vi "Chunk by Time.vi"(9 "Time Range (ns)":i64 format="%.0e", 10 "Max Frames":i32=1, 11 "Bytes in":u8[](array[numeric])) -> (2 "Chunks":T1[](array[typedef]), 3 "Bytes out":u8[](array[numeric]))   [LabVIEW 2021, in "pcap_Parse_Build_CIF.lvclass"]
doc: "Update all timestamps in the pcap bytestream. This will automatically detect if a global header is present and will work on both full pcap streams to/from disk and pcap packets to/from FIFO. If no global header is found it will default to CIF channel format (little endian, ns timestamp)."
uses:
  pcap_Parse_Build_CIF.lvclass
  Typedef/Chunk.ctl
  pcap_Parse_Build_CIF.lvclass/pcap_Parse_Build_CIF.ctl
  Parse/Unflatten Packet Header.vi
  Add Error.vi
  <vilib>/CIF Foundation/CIF Utilities/DataTypes/Flatten Unflatten/Unflatten U32.vi
  <vilib>/CIF Foundation/CIF Utilities/Errors/Append Error Location.vi
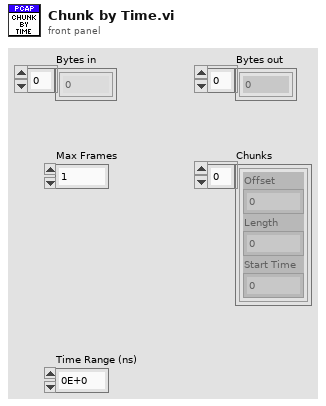
[diagram p1: front panel]
types:
  T1 = typedef "pcap_Parse_Build_CIF.lvclass/Chunk.ctl" = cluster{"Offset":i32, "Length":u32, "Start Time":i64}
  T2 = typedef "pcap_Parse_Build_CIF.lvclass/Packet Header.ctl" = cluster{"Timestamp (s)":u32, "Timestamp (ns)":u32, "Inc Length":u32, "Orig Length":u32}
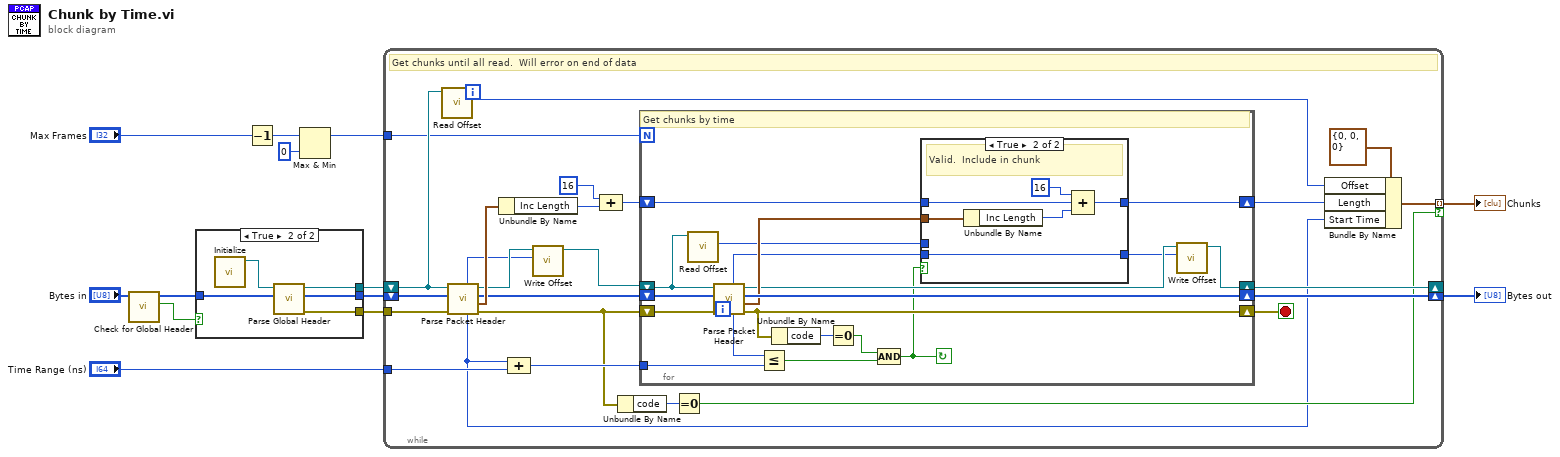
[diagram p0: block diagram]
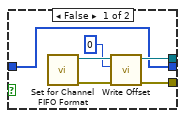
[diagram p2: hidden frame]
diagram:
  n1 = call "Check for Global Header.vi"("Bytes in"="Bytes in") -> ("Global Header Present"=w12:bool, "Bytes out"=w13:u8[])  [unwired: 8 in, 1 out]
  n2 = case shown="True" w12 {
    tunnel: [w16 w20] -> w1
    tunnel: w13 -> [w14 w23]
    tunnel: [w14 w22] -> w2
    tunnel: [w18 w21] -> w11
    frame False {
      n3 = call "Set for Channel FIFO Format.vi"() -> ("error out"=w18:errorcluster, "pcap_Parse_Build_CIF out"=w17:refnum<class "pcap_Parse_Build_CIF.lvclass">)  [unwired: 10 in]
      n4 = call "Write Offset.vi"("Offset"=0, "pcap Parse and Build in"=w17) -> ("pcap Parse and Build out"=w16:refnum<class "pcap_Parse_Build_CIF.lvclass">)  [unwired: 8 in, 1 out]
    }
    frame True {
      n5 = call "Initialize.vi"() -> ("pcap Parse and Build out"=w19:refnum<class "pcap_Parse_Build_CIF.lvclass">)  [unwired: 11 in]
      n6 = call "Parse Global Header.vi"("Bytes in"=w23, "pcap Parse and Build in"=w19) -> ("error out"=w21:errorcluster, "Bytes out"=w22:u8[], "pcap Parse and Build out"=w20:refnum<class "pcap_Parse_Build_CIF.lvclass">)  [unwired: 6 in, 1 out]
    }
  }
  n7 = Decrement(x="Max Frames") -> (x-1=w10:i32)
  n8 = Max & Min(x=w10, y=0) -> (max(x,y)=w9:i32)  [unwired: 1 out]
  n9 = while {
    tunnel: w9 -> [w44]
    tunnel: w11 -> [w47]
    tunnel: "Time Range (ns)" -> [w45]
    shift-right: [w38] -> w5
    shift-left: w2 -> [w48]
    shift-right: [w37] -> _
    shift-left: w1 -> [w46]
    tunnel: [w36] -> w4 mode=indexing if=w33
    stop <- w39 stop-if-true
    # "Get chunks until all read.  Will error on end of data"
    n10 = call "Read Offset.vi"("pcap Parse and Build in"=w46) -> ("Offset"=w31:i32)  [unwired: 8 in, 2 out]
    n11 = call "Parse Packet Header.vi"("error in (no error)"=w47, "Bytes in"=w48, "pcap Parse and Build in"=w46) -> ("error out"=w32:errorcluster, "Packet Header"=w43:T2, "Bytes out"=w41:u8[], "pcap Parse and Build out"=w30:refnum<class "pcap_Parse_Build_CIF.lvclass">, "TAI Time (ns)"=w24:i64, "Next Packet offset"=w28:i32)  [unwired: 3 in]
    n12 = Unbundle By Name(w43) -> ("Inc Length"=w27:u32)
    n13 = Compound Arithmetic op=ADD(w24, w45) -> (w42:i64)
    n14 = call "Write Offset.vi"("Offset"=w28, "pcap Parse and Build in"=w30) -> ("pcap Parse and Build out"=w29:refnum<class "pcap_Parse_Build_CIF.lvclass">)  [unwired: 8 in, 1 out]
    n15 = Compound Arithmetic op=ADD(u32 16 ("value"), w27) -> (w25:u32)
    n16 = Unbundle By Name(w32) -> ("code"=w34:i32)
    n17 = for {
      N: w44 -> [_]
      shift-right: [w54] -> w37
      shift-left: w29 -> [w58]
      shift-right: [w64] -> w38
      shift-left: w41 -> [w67]
      tunnel: w42 -> [w63]
      shift-right: [w50] -> w40
      shift-left: w25 -> [w53]
      shift-right: [w59] -> w39
      shift-left: w32 -> [w66]
      stop <- w51 continue-if-true
      # "Get chunks by time"
      n18 = call "Read Offset.vi"("pcap Parse and Build in"=w58) -> ("Offset"=w52:i32)  [unwired: 8 in, 2 out]
      n19 = call "Parse Packet Header.vi"("error in (no error)"=w66, "Bytes in"=w67, "pcap Parse and Build in"=w58) -> ("error out"=w59:errorcluster, "Packet Header"=w61:T2, "Bytes out"=w64:u8[], "pcap Parse and Build out"=w55:refnum<class "pcap_Parse_Build_CIF.lvclass">, "TAI Time (ns)"=w62:i64, "Next Packet offset"=w56:i32)  [unwired: 3 in]
      n20 = Less Or Equal?(x=w62, y=w63) -> (x <= y?=w57:bool)
      n21 = Unbundle By Name(w59) -> ("code"=w65:i32)
      n22 = Equal To 0?(x=w65) -> (x = 0?=w60:bool)
      n23 = Compound Arithmetic op=AND(w60, w57) -> (w51:bool)
      n24 = case shown="True" w51 {
        tunnel: w61 -> [_ w75]
        tunnel: w53 -> [w69 w74]
        tunnel: [w69 w72] -> w50
        tunnel: w52 -> [w68 _]
        tunnel: w56 -> [_ w71]
        tunnel: [w68 w71] -> w49
        frame False {
          # "Time not valid, don't include and revert offset."
        }
        frame True {
          # "Valid.  Include in chunk"
          n25 = Unbundle By Name(w75) -> ("Inc Length"=w73:u32)
          n26 = Compound Arithmetic op=ADD(u32 16 ("value"), w74, w73) -> (w72:u32)
        }
      }
      n27 = call "Write Offset.vi"("Offset"=w49, "pcap Parse and Build in"=w55) -> ("pcap Parse and Build out"=w54:refnum<class "pcap_Parse_Build_CIF.lvclass">)  [unwired: 8 in, 1 out]
    }
    n28 = Equal To 0?(x=w34) -> (x = 0?=w33:bool)
    n29 = Bundle By Name(cluster=T1 {"Offset"=0, "Length"=0, "Start Time"=0} ("Chunk"), "Offset"=w31, "Length"=w40, "Start Time"=w24) -> (w36:T1)
  }
  "Bytes out" <- w5
  "Chunks" <- w4
